vi "Close exe panel.vi"(8 "error in":errorcluster, 11 "VI ref":refnum<vi>) -> (0 "error out":errorcluster)   [LabVIEW 2020]
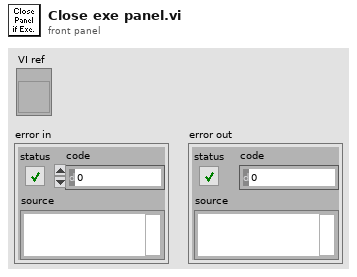
[diagram p1: front panel]
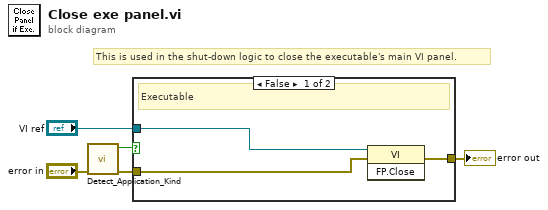
[diagram p0: block diagram]
diagram:
  # "This is used in the shut-down logic to close the executable's main VI panel."
  n1 = call <userlib>:"Detect_Application_Kind.vi"("error in"="error in") -> ("error out"=w4:errorcluster, "Development System"=w5:bool)  [unwired: 8 in, 1 out]
  n2 = case shown="False" w5 {
    tunnel: w4 -> [w8 w9]
    tunnel: [w7 w9] -> w3
    tunnel: "VI ref" -> [w6 _]
    frame False {
      # "Executable"
      n3 = invoke class="VI" method="FP.Close"(reference=w6, error in=w8) -> (error out=w7:errorcluster)  [unwired: 1 in, 2 out]
    }
    frame True {
      # "Source code"
    }
  }
  "error out" <- w3
